vi "重构模块.vi"(0 "光源实数二维数组":dbl[][](array[numeric]), 1 "物体1024一维数组":dbl[](array[numeric]), 2 "重建方法":u16(ring) items=["二阶重构", "压缩感知"], 3 "光源二维数组列平均值":dbl[](array[numeric]), 4 "采样次数":i32, 5 "正图像筛选门限":dbl) -> (14 "重构图像":dbl[][](array[numeric]))   [LabVIEW 2018]
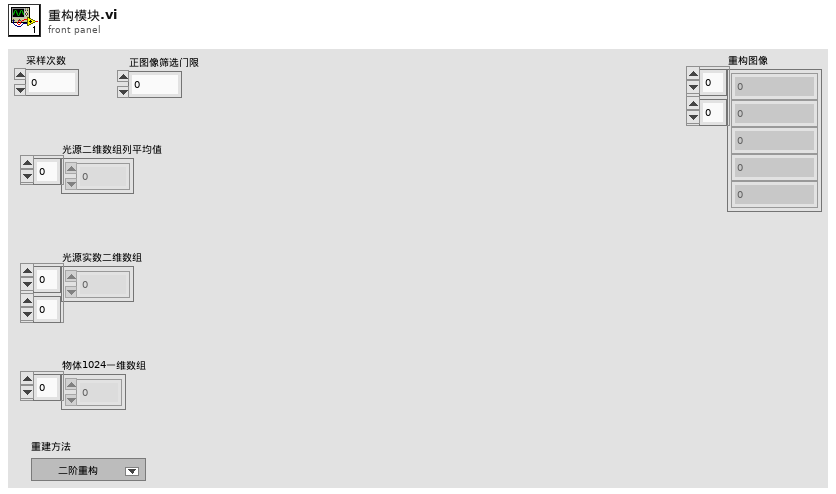
[diagram p1: front panel]
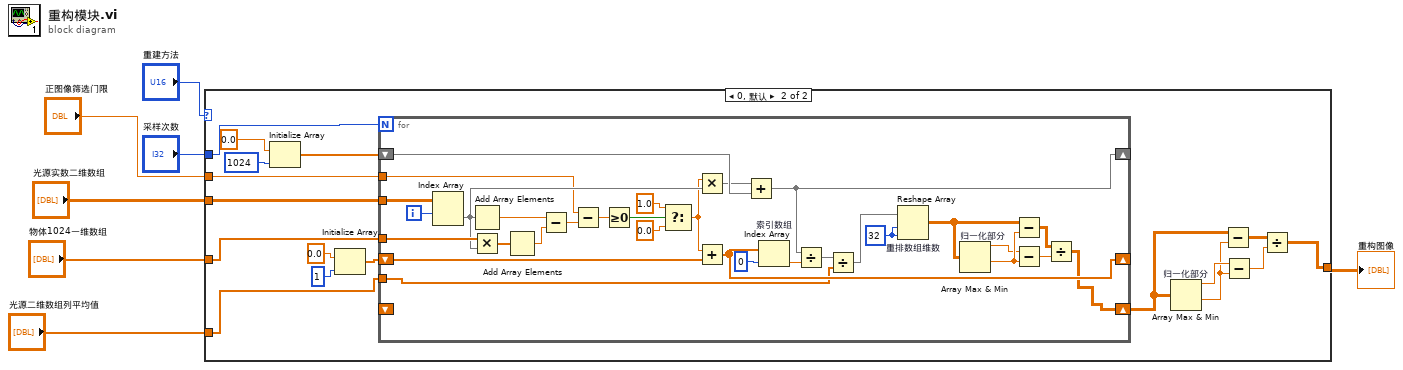
[diagram p0: block diagram]
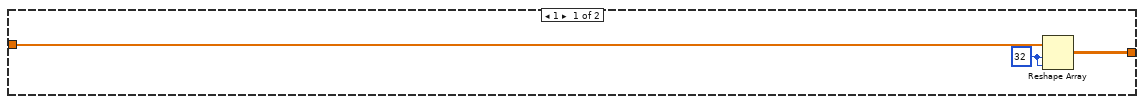
[diagram p2: hidden frame]
diagram:
  n1 = case shown="0, 默认" "重建方法" {
    tunnel: "采样次数" -> [_ w27]
    tunnel: "光源实数二维数组" -> [_ w24]
    tunnel: "物体1024一维数组" -> [w9 w21]
    tunnel: [w8 w12] -> w6
    tunnel: "正图像筛选门限" -> [_ w17]
    tunnel: "光源二维数组列平均值" -> [_ w18]
    frame 1 {
      w10 = 32
      n2 = Reshape Array(w9, w10, w10) -> (w8:dbl[][])
    }
    frame 0, Default {
      n3 = Initialize Array(0.0 ("元素"), 1024 ("维数大小")) -> (w20:dbl[])
      n4 = Initialize Array(0.0 ("元素"), 1 ("维数大小")) -> (w19:dbl[])
      n5 = for {
        N: w27 -> [_]
        tunnel: w24 -> [w57]
        tunnel: w21 -> [w56]
        shift-right: [w43] -> _
        shift-left: w20 -> [w47]
        shift-right: [w39] -> _
        shift-left: w19 -> [w41]
        tunnel: w17 -> [w35]
        tunnel: w18 -> [w29]
        shift-right: [w28] -> w11
        shift-left: _ -> [_]
        i -> [w58]
        w50 = 32 ("维数大小")
        n6 = Index Array(array=w57, index (row)=w58) -> (element=w44:dbl[])  [unwired: 1 in]
        n7 = Add Array Elements(numeric array=w44) -> (sum=w38:dbl)
        n8 = Multiply(x=w56, y=w44) -> (x*y=w55:dbl[])
        n9 = Add Array Elements(numeric array=w55) -> (sum=w37:dbl)
        n10 = Subtract(x=w38, y=w37) -> (x-y=w36:dbl)
        n11 = Subtract(x=w35, y=w36) -> (x-y=w34:dbl)
        n12 = Greater Or Equal To 0?(x=w34) -> (x >= 0?=w31:bool)
        n13 = Select(t=1.0, s=w31, f=0.0) -> (s? t:f=w30:dbl)
        n14 = Multiply(x=w30, y=w44) -> (x*y=w45:dbl[])
        n15 = Add(x=w30, y=w41) -> (x+y=w39:dbl[])
        n16 = Add(x=w45, y=w47) -> (x+y=w43:dbl[])
        n17 = Index Array "索引数组"(array=w39, index=0 ("索引")) -> (element=w40:dbl)
        n18 = Divide(x=w43, y=w40) -> (x/y=w46:dbl[])
        n19 = Divide(x=w46, y=w29) -> (x/y=w48:dbl[])
        n20 = Reshape Array "重排数组维数"(w48, w50, w50) -> (w49:dbl[][])
        n21 = Array Max & Min "归一化部分"(array=w49) -> (max value=w51:dbl, min value=w52:dbl)  [unwired: 2 out]
        n22 = Subtract(x=w49, y=w52) -> (x-y=w53:dbl[][])
        n23 = Subtract(x=w51, y=w52) -> (x-y=w54:dbl)
        n24 = Divide(x=w53, y=w54) -> (x/y=w28:dbl[][])
      }
      n25 = Array Max & Min "归一化部分"(array=w11) -> (max value=w16:dbl, min value=w15:dbl)  [unwired: 2 out]
      n26 = Subtract(x=w11, y=w15) -> (x-y=w14:dbl[][])
      n27 = Subtract(x=w16, y=w15) -> (x-y=w13:dbl)
      n28 = Divide(x=w14, y=w13) -> (x/y=w12:dbl[][])
    }
  }
  "重构图像" <- w6
